vi "saveTimeSeries.vi"(0 "1":dbl, 1 "save?":bool, 2 "Number of Data Series":enum16{"1", "2", "3", "4"}(ring), 5 "2":dbl, 7 "3":dbl, 9 "4":dbl, 11 "Error In":errorcluster, 12 "file path (dialog if empty)":path) -> (15 "Error Out":errorcluster)   [LabVIEW 2011]
uses:
  <vilib>/Utility/file.llb/Write To Spreadsheet File (string).vi
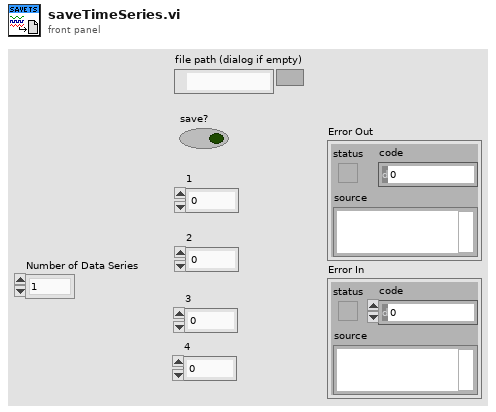
[diagram p1: front panel]
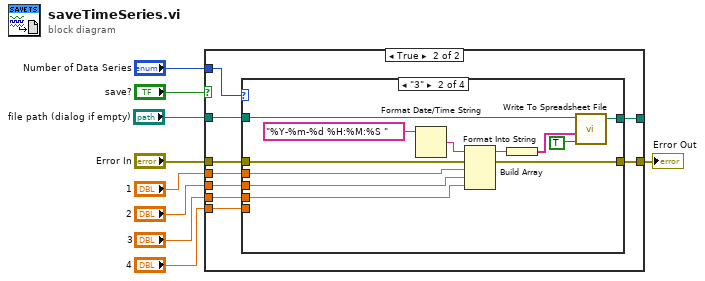
[diagram p0: block diagram]
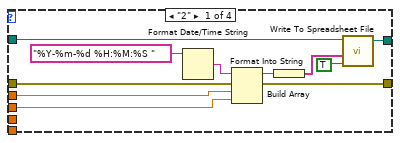
[diagram p3: hidden frame]
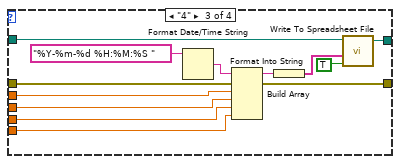
[diagram p4: hidden frame]
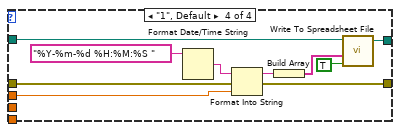
[diagram p5: hidden frame]
diagram:
  n1 = case shown="True" "save?" {
    tunnel: "3" -> [_ w20]
    tunnel: "2" -> [_ w19]
    tunnel: "1" -> [_ w18]
    tunnel: "file path (dialog if empty)" -> [w11 w17]
    tunnel: [w11 w16] -> _
    tunnel: "Error In" -> [w10 w15]
    tunnel: [w10 w14] -> w2
    tunnel: "4" -> [_ w13]
    tunnel: "Number of Data Series" -> [_ w12]
    frame False {
    }
    frame True {
      n2 = case shown="\"3\"" w12 {
        tunnel: w20 -> [_ w43 w56 _]
        tunnel: w19 -> [w31 w42 w55 _]
        tunnel: w18 -> [w30 w41 w54 w66]
        tunnel: w17 -> [w29 w40 w53 w65]
        tunnel: [w28 w39 w52 w64] -> w16
        tunnel: w15 -> [w22 w33 w46 w58]
        tunnel: [w21 w32 w45 w57] -> w14
        tunnel: w13 -> [_ _ w44 _]
        frame "2" {
          n3 = Format Date/Time String(time format string (%c)="%Y-%m-%d %H:%M:%S ") -> (date/time string=w26:string)  [unwired: 2 in]
          n4 = Format Into String(initial string=w26, error in=w22, w30, w31) -> (resulting string=w24:string, error out=w21:errorcluster)  [unwired: 1 in]
          n5 = Build Array(w24) -> (w23:string[])
          n6 = call-poly <vilib>:"Write To Spreadsheet File.vi"("append to file? (new file:F)"=TRUE, "1D data"=w23, "file path (dialog if empty)"=w29) -> ("new file path (Not A Path if cancelled)"=w28:path)  [unwired: 5 in]
        }
        frame "3" {
          n7 = Format Date/Time String(time format string (%c)="%Y-%m-%d %H:%M:%S ") -> (date/time string=w37:string)  [unwired: 2 in]
          n8 = Format Into String(initial string=w37, error in=w33, w41, w42, w43) -> (resulting string=w35:string, error out=w32:errorcluster)  [unwired: 1 in]
          n9 = Build Array(w35) -> (w34:string[])
          n10 = call-poly <vilib>:"Write To Spreadsheet File.vi"("append to file? (new file:F)"=TRUE, "1D data"=w34, "file path (dialog if empty)"=w40) -> ("new file path (Not A Path if cancelled)"=w39:path)  [unwired: 5 in]
        }
        frame "4" {
          n11 = Format Date/Time String(time format string (%c)="%Y-%m-%d %H:%M:%S ") -> (date/time string=w50:string)  [unwired: 2 in]
          n12 = Format Into String(initial string=w50, error in=w46, w54, w55, w56, w44) -> (resulting string=w48:string, error out=w45:errorcluster)  [unwired: 1 in]
          n13 = Build Array(w48) -> (w47:string[])
          n14 = call-poly <vilib>:"Write To Spreadsheet File.vi"("append to file? (new file:F)"=TRUE, "1D data"=w47, "file path (dialog if empty)"=w53) -> ("new file path (Not A Path if cancelled)"=w52:path)  [unwired: 5 in]
        }
        frame "1", Default {
          n15 = Format Date/Time String(time format string (%c)="%Y-%m-%d %H:%M:%S ") -> (date/time string=w62:string)  [unwired: 2 in]
          n16 = Format Into String(initial string=w62, error in=w58, w66) -> (resulting string=w60:string, error out=w57:errorcluster)  [unwired: 1 in]
          n17 = Build Array(w60) -> (w59:string[])
          n18 = call-poly <vilib>:"Write To Spreadsheet File.vi"("append to file? (new file:F)"=TRUE, "1D data"=w59, "file path (dialog if empty)"=w65) -> ("new file path (Not A Path if cancelled)"=w64:path)  [unwired: 5 in]
        }
      }
    }
  }
  "Error Out" <- w2
